vi "forloop.vi"() -> ()   [LabVIEW 2017]
panel:
  out "x+y":i32
  out "Gauge":dbl(knob) scale=0.0..1000.0
  out "Numeric":dbl
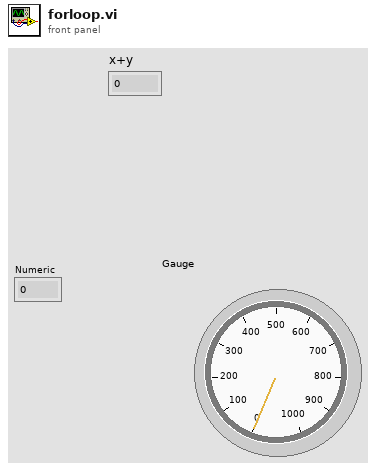
[diagram p1: front panel]
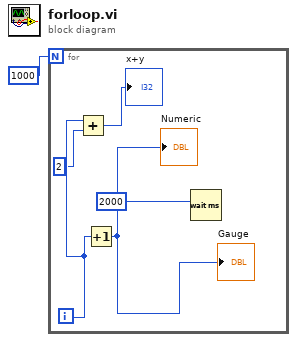
[diagram p0: block diagram]
diagram:
  n1 = for {
    N: 1000 -> [_]
    i -> [w4]
    n2 = Add(x=w4, y=2) -> (x+y=→"x+y":i32)
    n3 = Increment(x=w4) -> (x+1=→"Numeric" →"Gauge":i32)
    n4 = Wait (ms)(milliseconds to wait=u32 2000 ("millisecond timer value")) -> ()  [unwired: 1 out]
  }
